vi "OCR_Find FG and BG.vi"(8 "Letter Color Array":T1={"BG"=239, "FG"=65793}, 11 "Current BG Color":u32(colorbox)) -> (3 "Color Set":T1={"BG"=239, "FG"=65793})   [LabVIEW 2009]
uses:
  Controls/Cluster/Cluster_Text Color Set.ctl
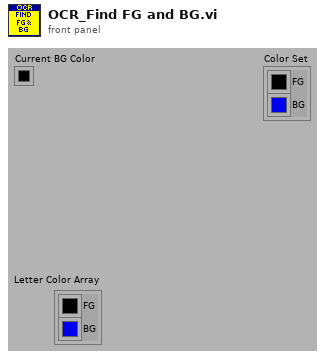
[diagram p1: front panel]
types:
  T1 = typedef "Cluster_Text Color Set.ctl" = cluster{"BG":u32, "FG":u32}
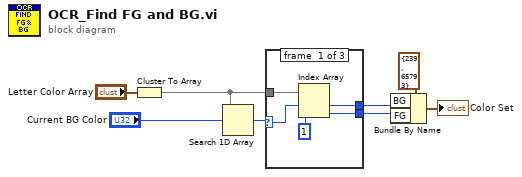
[diagram p0: block diagram]
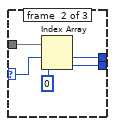
[diagram p2: hidden frame]
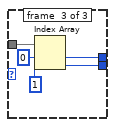
[diagram p3: hidden frame]
diagram:
  n1 = Cluster To Array(cluster="Letter Color Array") -> (array=w1:u32[])
  n2 = Search 1D Array(1D array=w1, element="Current BG Color") -> (index of element=w2:i32)  [unwired: 1 in]
  n3 = case shown="1.." w2 {
    selector: w2 -> [w12 w17 _]
    tunnel: w1 -> [w13 w18 w23]
    tunnel: [w10 w15 w20] -> w4
    tunnel: [w9 w14 w19] -> w3
    frame #0 {
      n4 = Index Array(array=w13, index #1=w12, index #2=1 ("index")) -> (element #1=w10:u32, element #2=w9:u32)
    }
    frame #1 {
      n5 = Index Array(array=w18, index #1=w17, index #2=0 ("index")) -> (element #1=w15:u32, element #2=w14:u32)
    }
    frame #2 {
      n6 = Index Array(array=w23, index #1=0 ("index"), index #2=1 ("index")) -> (element #1=w20:u32, element #2=w19:u32)
    }
  }
  n7 = Bundle By Name(cluster=T1 {"BG"=239, "FG"=65793} ("Color Set"), "BG"=w4, "FG"=w3) -> (→"Color Set":T1)
